vi "Server TLS Config Control.vi"() -> ()   [LabVIEW 2020]
uses:
  TCP Comms/Cert Chain.ctl
  TCP Comms/TinyTCP.lvlib
  TCP Comms/Server TLS Config.ctl
panel:
  in  "Server TLS Config":T1
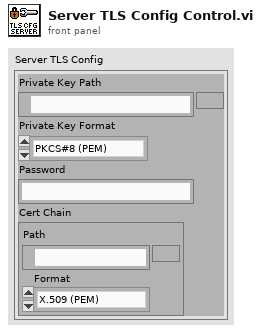
[diagram p1: front panel]
types:
  T1 = typedef "TinyTCP.lvlib/Server TLS Config.ctl" = cluster{"Private Key Path":path, "Private Key Format":enum32{"PKCS#8 (PEM)", "PKCS#8 (DER)"}, "Password":string, "Cert Chain":T2}
  T2 = typedef "TinyTCP.lvlib/Cert Chain.ctl" = cluster{"Path":path, "Format":enum32{"X.509 (PEM)"}}
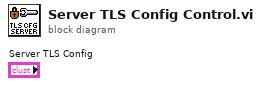
[diagram p0: block diagram]
diagram:
